vi "Float CNV.vi"(7 "精度(6)":i16, 11 "数值":sgl) -> (3 "字符串":string)   [LabVIEW 2016, in "DGUS.lvlib" / "DGUS.lvclass"]
uses:
  DGUS.lvclass
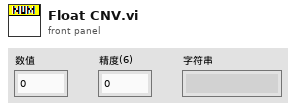
[diagram p1: front panel]
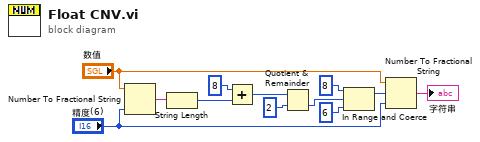
[diagram p0: block diagram]
diagram:
  n1 = Number To Fractional String(number="数值", precision (6)="精度(6)") -> (F-format string=w12:string)  [unwired: 2 in]
  n2 = String Length(string=w12) -> (length=w7:i32)
  n3 = Add(x=8, y=w7) -> (x+y=w6:i32)
  n4 = Quotient & Remainder(x=w6, y=2) -> (floor(x/y)=w4:i32)  [unwired: 1 out]
  n5 = In Range and Coerce(upper limit=8 ("上限"), x=w4, lower limit=6 ("下限")) -> (coerced(x)=w1:i32)  [unwired: 1 out]
  n6 = Number To Fractional String(number="数值", width (-)=w1, precision (6)="精度(6)") -> (F-format string=→"字符串":string)  [unwired: 1 in]
